vi "configuration UI.vi"() -> ()   [LabVIEW 2013, in "configuration tests.lvlib" / "TEST EDITOR.lvclass"]
uses:
  TEST EDITOR.lvclass
  <vilib>/NI/Configuration Framework/Node/NodeRef.ctl
  <vilib>/NI/Configuration Framework/Node/NISE_CEF_Node.lvclass
  <vilib>/NI/AMC/Message Queue.ctl
  <vilib>/NI/AMC/Message.ctl
  <vilib>/NI/Tools/Keyed Array/KeyedArray.ctl
  <vilib>/NI/Configuration Framework/Node/UserEventRef.ctl
  <vilib>/NI/Configuration Framework/Controls/EventCluster.ctl
  module/configuration/TEST CONFIGURATION.lvclass
  TEST EDITOR.lvclass/TEST EDITOR.ctl
  <vilib>/NI/Configuration Framework/serializable configuration/NISE_CEF_serializable configuration.lvclass/NISE_CEF_serializable configuration.ctl
  Configuration Editor/Classes/Engine Parent/Engine Parent Editor Node.lvclass
  module/configuration/TEST CONFIGURATION.lvclass/TEST CONFIGURATION.ctl
  module/configuration/gains.ctl
  Read sort_.vi
  module/configuration/Read state module configuration.vi
  Write sort_.vi
  <vilib>/NI/Configuration Framework/serializable configuration/Read UID.vi
  Configuration Editor/Classes/Module editor node/Read Module Configuration.vi
  <vilib>/Utility/LVClass/Get LV Class Name.vi
  <vilib>/NI/Configuration Framework/error generator/NISE_error generator.vi
  <vilib>/NI/Tag Bus Module Framework/module configuration/TBM module configuration.lvclass
  <vilib>/NI/Tag Bus Module Framework/channel/TBM channel.lvclass
  <vilib>/NI/Configuration Framework/NISE_CEF_TreeControl.lvlib
  <vilib>/NI/Tools/Keyed Array/Tools_KeyedArray.lvlib
  <vilib>/NI/AMC/AMC.lvlib
panel:
  in  "Tab Control":T1(tab)
  in  "delete":bool
  in  "add":bool
  in  "Result Tag":u16(ring)
  in  "PV Tag":u16(ring)
  in  "Setpoint Tag":u16(ring)
  in  "Functions":i32(listbox)
  in  "Function Name":string
  in  "Lower Limit":dbl=-100.0
  in  "Upper Limit":dbl=100.0
  in  "Ki":dbl
  in  "Kd":dbl
  in  "Kp":dbl
  in  "Output Tag":u16(ring)
  in  "Input Tag":u16(ring)
  in  "user event":T2
  in  "main queue":T3
  in  "node ref":T4
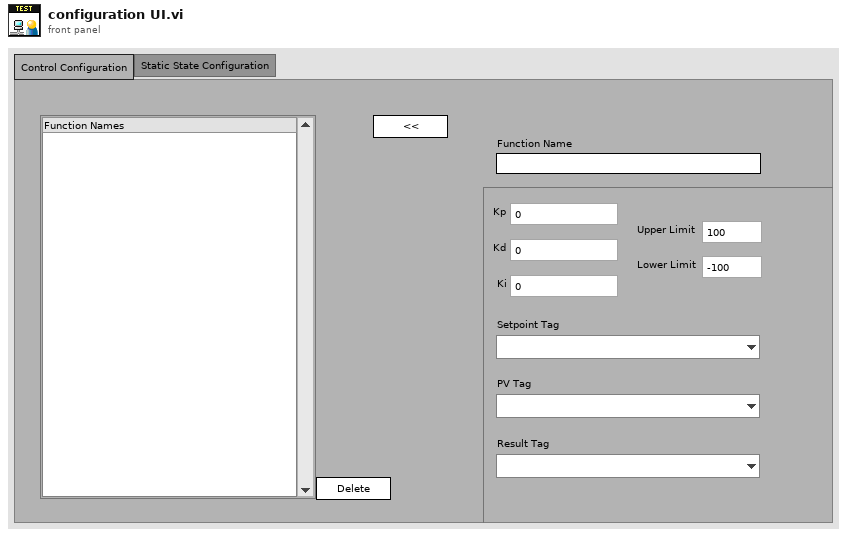
[diagram p1: front panel]
types:
  T1 = enum32{"Control Configuration", "Static State Configuration"}
  T2 = typedef "NISE_CEF_Node.lvclass/UserEventRef.ctl" = refnum<user-event>
  T3 = typedef "AMC.lvlib/Message Queue.ctl" = refnum<queue>
  T4 = typedef "NISE_CEF_Node.lvclass/NodeRef.ctl" = refnum<data-value>
  T5 = typedef "NISE_CEF_TreeControl.lvlib/EventCluster.ctl" = cluster{"command":string, "data":string}
  T6 = typedef "configuration tests.lvlib/TEST CONFIGURATION.lvclass/gains.ctl" = cluster{"Kp":dbl, "Ki":dbl, "Kd":dbl}
  T7 = typedef "user tag bus module configuration.lvclass/state module configuration.ctl" = cluster{"fixed input":refnum<class "TBM channel.lvclass">, "fixed output":refnum<class "TBM channel.lvclass">, "initial state":u8}
  T8 = typedef "configuration tests.lvlib/TEST CONFIGURATION.lvclass/control module configuration.ctl" = cluster{"name":string, "setpoint":refnum<class "TBM channel.lvclass">, "process variable":refnum<class "TBM channel.lvclass">, "output":refnum<class "TBM channel.lvclass">, "gains":T6, "output range":cluster{"output high":dbl, "output low":dbl}}
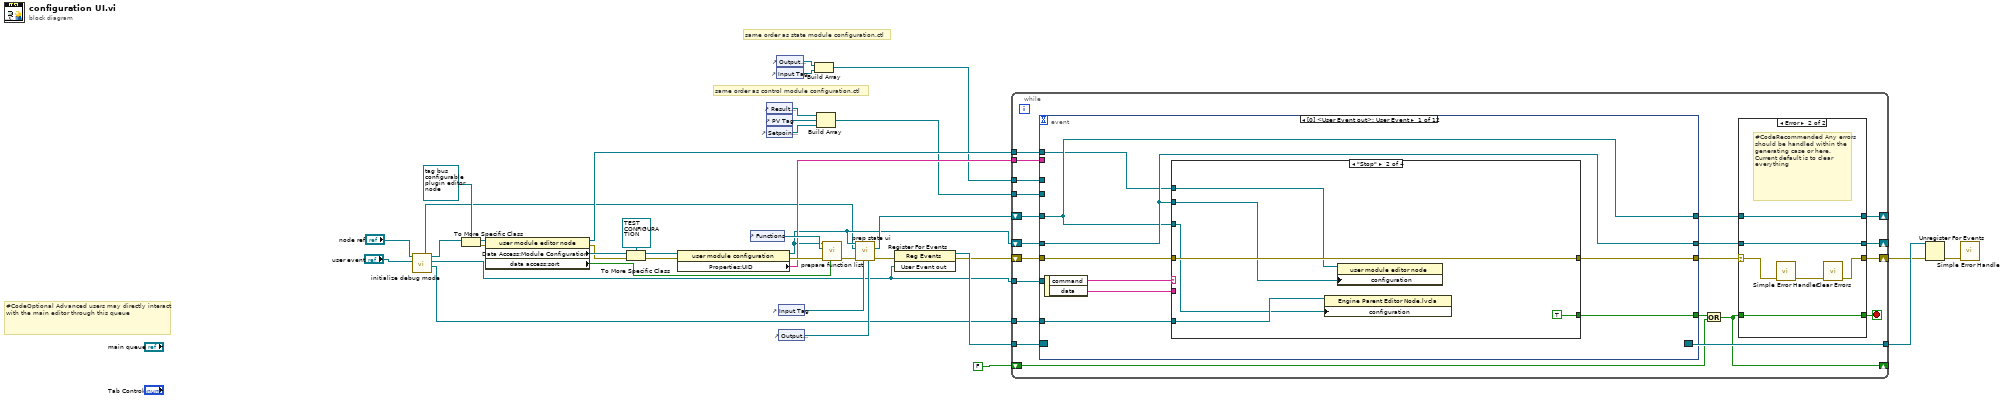
[diagram p0: block diagram]
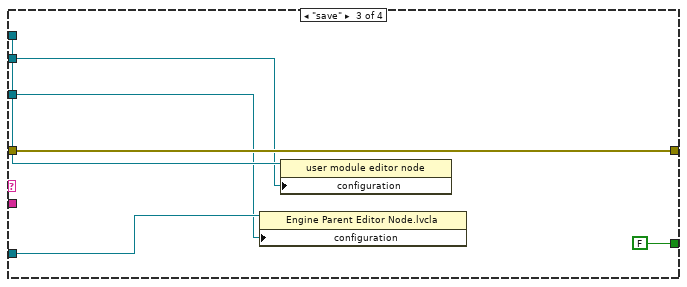
[diagram p4: hidden frame]
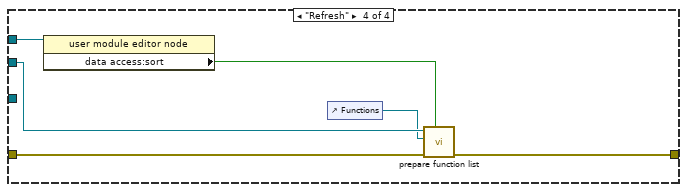
[diagram p5: hidden frame]
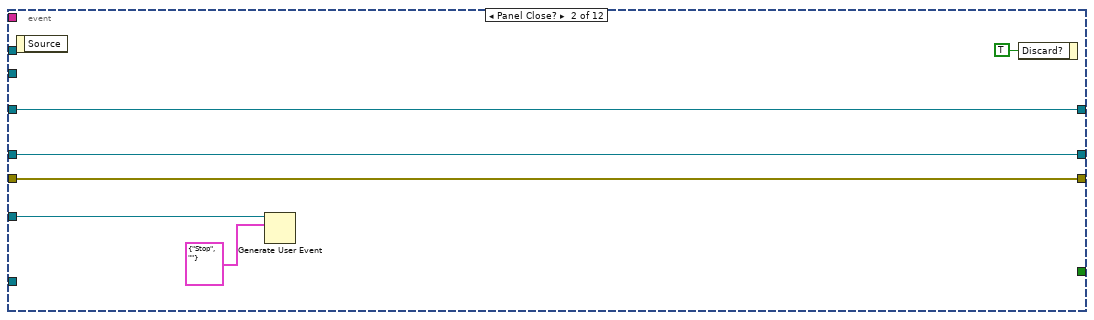
[diagram p6: hidden frame]
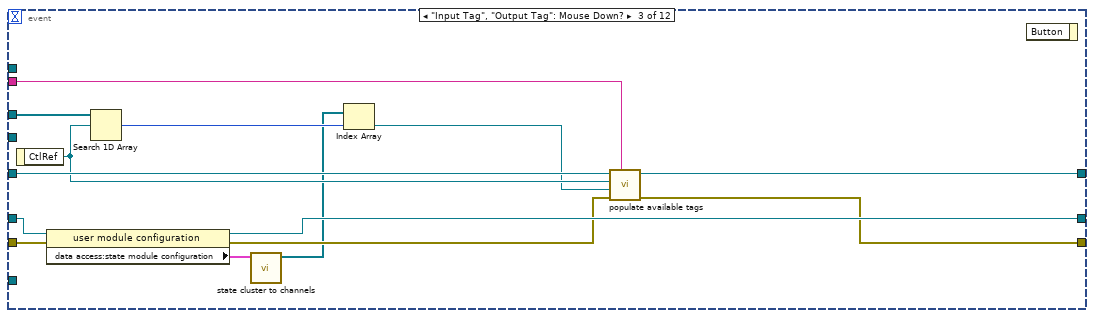
[diagram p7: hidden frame]
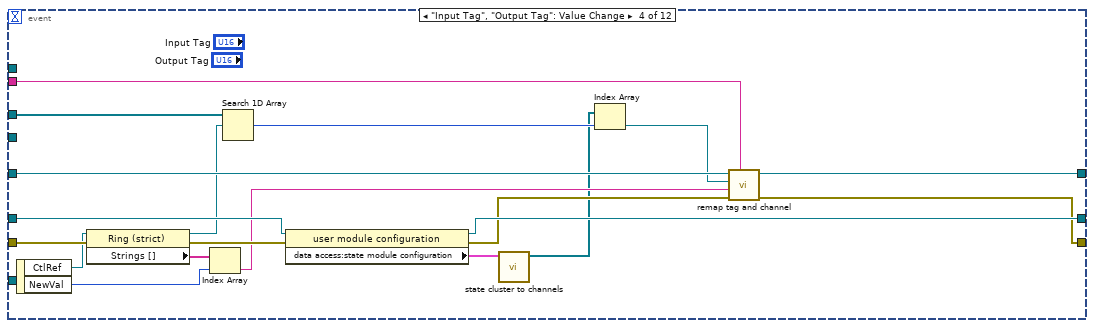
[diagram p8: hidden frame]
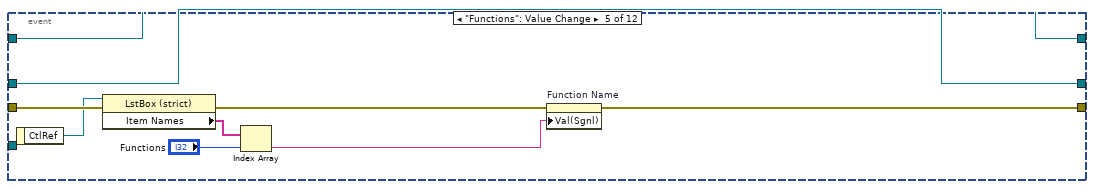
[diagram p9: hidden frame]
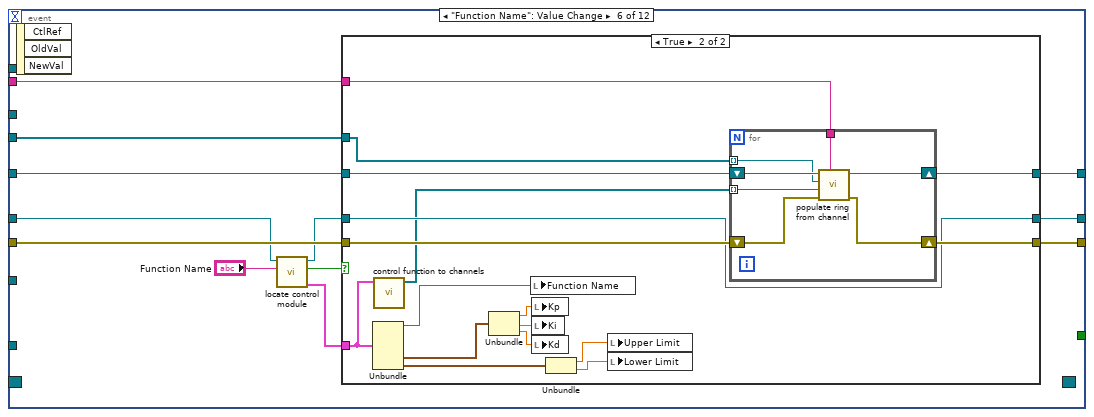
[diagram p10: hidden frame]
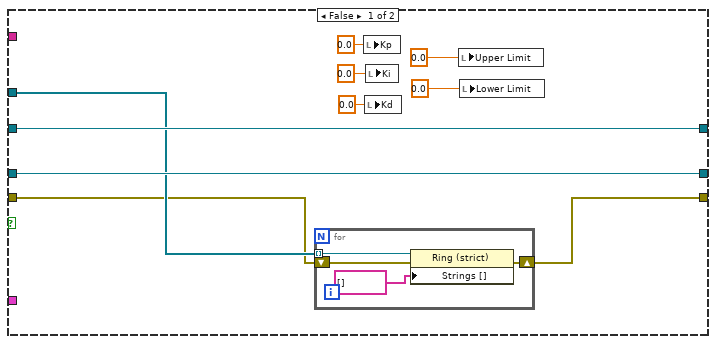
[diagram p11: hidden frame]
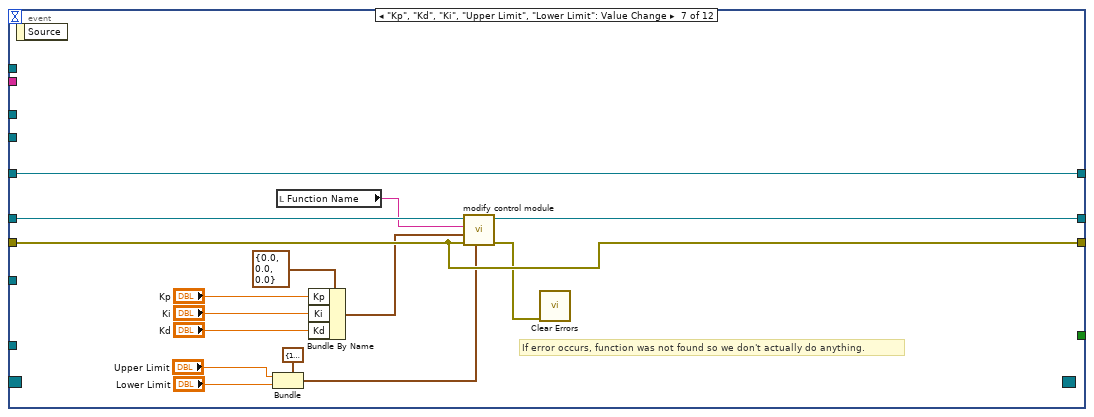
[diagram p12: hidden frame]
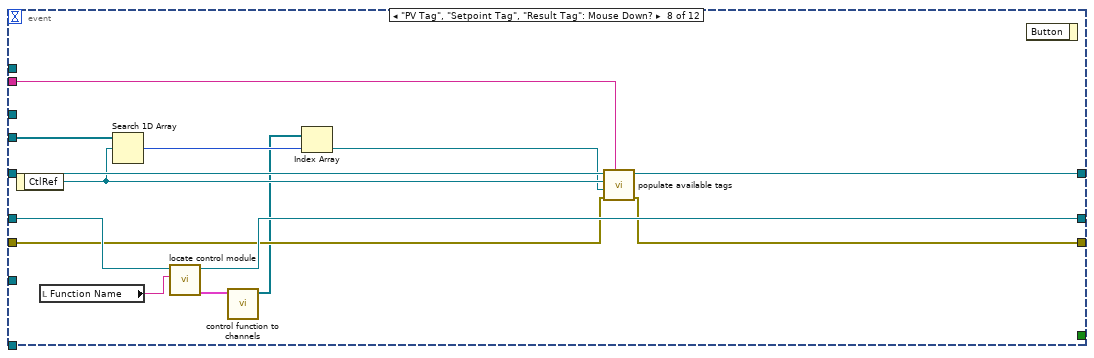
[diagram p13: hidden frame]
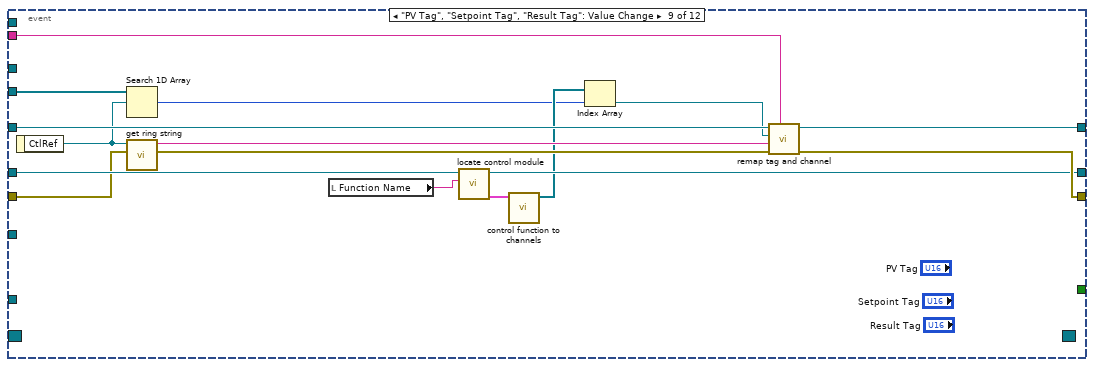
[diagram p14: hidden frame]
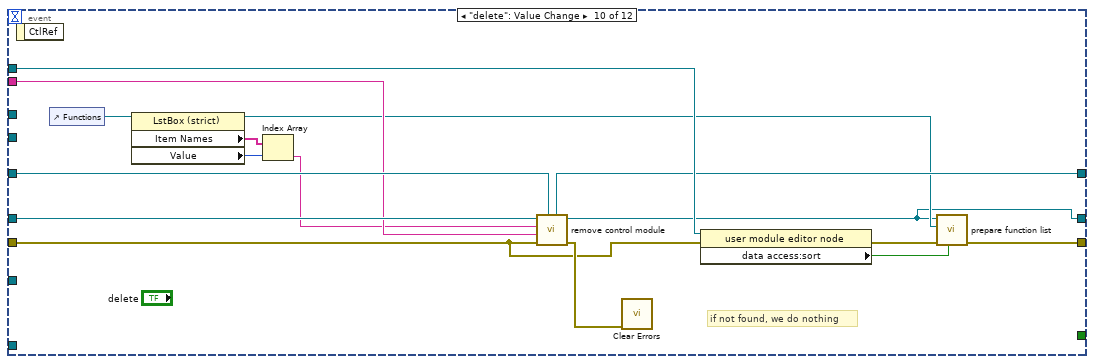
[diagram p15: hidden frame]
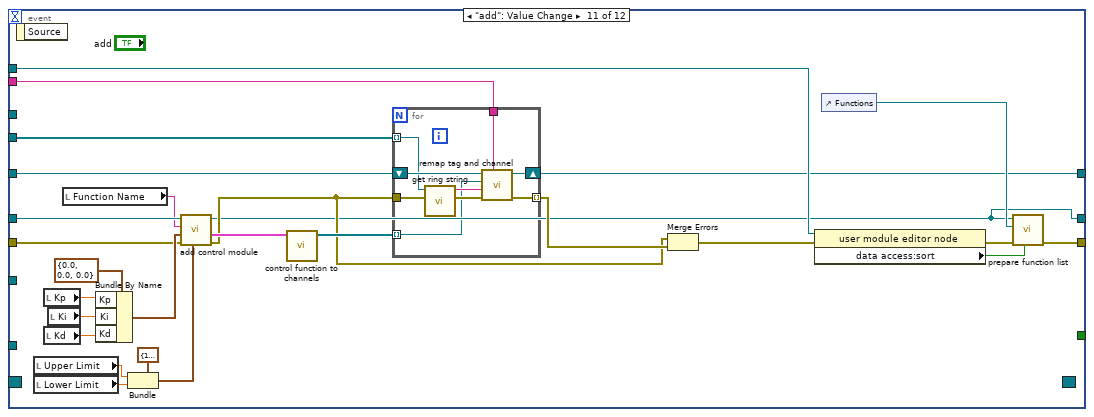
[diagram p16: hidden frame]
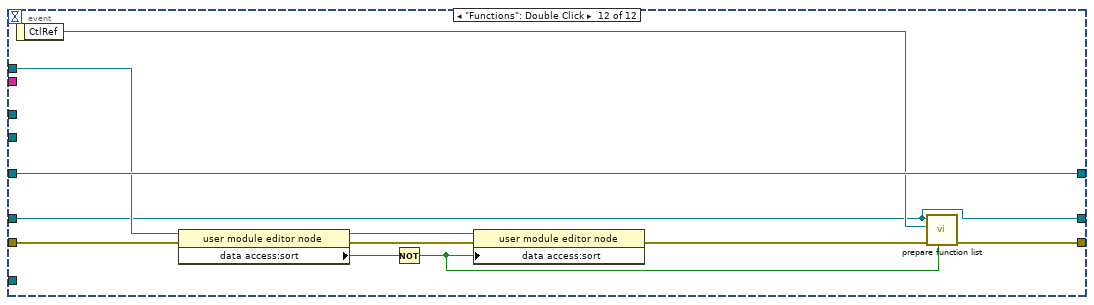
[diagram p17: hidden frame]
diagram:
  # "same order as control module configuration.ctl"
  # "same order as state module configuration.ctl"
  # "#CodeOptional Advanced users may directly interact with the main editor through this queue"
  n1 = call "initialize debug mode.vi"("User Event in"="user event", "editor node in"="node ref") -> ("engine"=w6:refnum<data-value>, "User Event out"=w1:T2, "editor node out"=w5:T4, "Engine Configuration"=w2:refnum<class "engine configuration.lvclass">)  [unwired: 6 in]
  n2 = To More Specific Class(target class=refnum<data-value> refnum ("data value reference"), reference=w5) -> (specific class reference=w31:refnum<data-value>, error out=w30:errorcluster)  [unwired: 1 in]
  n3 = property class="user module editor node"(reference=w31, error in=w30) -> (reference out=w16:refnum<data-value>, error out=w25:errorcluster, "Data Access:Module Configuration"=w29:refnum<class "TBM module configuration.lvclass">, "data access:sort"=w15:bool)
  n4 = To More Specific Class(target class=refnum<class "TEST CONFIGURATION.lvclass"> refnum ("user module configuration"), reference=w29, error in=w25) -> (specific class reference=w23:refnum<class "TEST CONFIGURATION.lvclass">, error out=w27:errorcluster)
  n5 = property class="user module configuration"(reference=w23, error in=w27) -> (reference out=w7:refnum<class "TEST CONFIGURATION.lvclass">, error out=w24:errorcluster, "Properties:UID"=w22:string)
  n6 = control-ref of="Functions"() -> (w26:refnum<vi>)
  n7 = control-ref of="Result Tag"() -> (w10:refnum<vi>)
  n8 = control-ref of="PV Tag"() -> (w12:refnum<vi>)
  n9 = control-ref of="Setpoint Tag"() -> (w11:refnum<vi>)
  n10 = control-ref of="Output Tag"() -> (w13:refnum<vi>)
  n11 = control-ref of="Input Tag"() -> (w14:refnum<vi>)
  n12 = control-ref of="Input Tag"() -> (w19:refnum<vi>)
  n13 = control-ref of="Output Tag"() -> (w18:refnum<vi>)
  n14 = Build Array(w13, w14) -> (w9:refnum<vi>[])
  n15 = Build Array(w10, w12, w11) -> (w8:refnum<vi>[])
  n16 = call "prepare function list.vi"("sort?"=w15, "error in"=w24, "Functions listbox"=w26, "configuration in"=w7) -> ("error out"=w20:errorcluster)  [unwired: 5 in]
  n17 = call "prep state ui.vi"("Output Tag"=w18, "Input Tag"=w19, "error in"=w20, "engine configuration in"=w2, "user tag bus module configuration in"=w7) -> ("error out"=w21:errorcluster, "engine configuration out"=w17:refnum<class "engine configuration.lvclass">)  [unwired: 5 in]
  n18 = register-events(error in=w21, w1) -> (reference out=w38:refnum<event-registration>, error out=w33:errorcluster)  [unwired: 1 in]
  n19 = while {
    tunnel: w38 -> [w59]
    tunnel: [w58] -> w37
    shift-right: [w51] -> w36
    shift-left: w33 -> [w57]
    shift-right: [w53] -> _
    shift-left: FALSE -> [w52]
    shift-right: [w48] -> _
    shift-left: w7 -> [w50]
    shift-right: [w45] -> _
    shift-left: w17 -> [w47]
    tunnel: w22 -> [w44]
    tunnel: w16 -> [w43]
    tunnel: w6 -> [w42]
    tunnel: w9 -> [w41]
    tunnel: w8 -> [w40]
    tunnel: w1 -> [w39]
    stop <- w55 stop-if-true
    n20 = event shown="[0] <User Event out>: User Event" {
      selector: w59 -> [_ _ _ _ _ _ _ _ _ _ _ _]
      dyn-events: [_ _ _ _ _ _ _ _ _ _ _ _] -> w58
      timeout: _ -> [_ _ _ _ _ _ _ _ _ _ _ _]
      tunnel: [w76 _ _ _ _ _ _ _ _ _ _ _] -> w54
      tunnel: [w77 w103 w113 w128 w137 w153 w209 w217 w238 w254 w283 w302] -> w56
      tunnel: w57 -> [w78 w103 w117 w136 w145 w157 w209 w218 w231 w251 w265 w301]
      tunnel: [w74 w102 w114 w130 w144 w154 w207 w223 w234 w241 w257 w293] -> w49
      tunnel: w50 -> [w74 w102 w115 w131 w144 w152 w210 w224 w235 w256 w275 w293]
      tunnel: w47 -> [w73 w101 w112 w133 w143 w155 w205 w221 w240 w248 w276 w303]
      tunnel: [w73 w101 w116 w129 w143 w156 w205 w220 w239 w247 w277 w303] -> w46
      tunnel: w44 -> [_ _ w111 w126 _ w148 _ w219 w237 w246 w278 _]
      tunnel: w43 -> [w72 _ _ _ _ _ _ _ _ w249 w279 w297]
      tunnel: w42 -> [w71 _ _ _ _ _ _ _ _ _ _ _]
      tunnel: w41 -> [_ _ w109 w124 _ _ _ _ _ _ _ _]
      tunnel: w40 -> [_ _ _ _ _ w146 _ w215 w230 _ w260 _]
      tunnel: w39 -> [_ w99 _ _ _ _ _ _ _ _ _ _]
      event User Event {
        n21 = event-data() -> ("command"=w75:string, "data"=w70:string)  [unwired: 1 in]
        n22 = case shown="\"Stop\"" w75 {
          tunnel: [_ TRUE FALSE _] -> w76
          tunnel: w71 -> [_ w84 w90 _]
          tunnel: w74 -> [_ w81 w86 w94]
          tunnel: w73 -> [_ w80 w87 _]
          tunnel: w78 -> [w79 w83 w89 w95]
          tunnel: [w79 w83 w89 w96] -> w77
          tunnel: w72 -> [_ w82 w88 w97]
          tunnel: w70 -> [_ _ _ _]
          frame Default {
          }
          frame "Stop" {
            n23 = property class="Engine Parent Editor Node.lvcla"(reference=w84, "configuration"=w80) -> ()  [unwired: 1 in, 2 out]
            n24 = property class="user module editor node"(reference=w82, "configuration"=w81) -> ()  [unwired: 1 in, 2 out]
          }
          frame "save" {
            n25 = property class="Engine Parent Editor Node.lvcla"(reference=w90, "configuration"=w87) -> ()  [unwired: 1 in, 2 out]
            n26 = property class="user module editor node"(reference=w88, "configuration"=w86) -> ()  [unwired: 1 in, 2 out]
          }
          frame "Refresh" {
            n27 = property class="user module editor node"(reference=w97) -> ("data access:sort"=w93:bool)  [unwired: 1 in, 2 out]
            n28 = control-ref of="Functions"() -> (w92:refnum<vi>)
            n29 = call "prepare function list.vi"("sort?"=w93, "error in"=w95, "Functions listbox"=w92, "configuration in"=w94) -> ("error out"=w96:errorcluster)  [unwired: 5 in]
          }
        }
      }
      event Panel Close? {
        n30 = event-data() -> ()  [unwired: 1 in, 1 out]
        n31 = Generate User Event(user event=w99, event data cluster=T5 {"command"="Stop", "data"=""} ("event data")) -> ()  [unwired: 2 in, 2 out]
        n32 = event-data("Discard?"=TRUE) -> ()  [unwired: 1 in, 1 out]
      }
      event "Input Tag", "Output Tag": Mouse Down? {
        n33 = event-data() -> ("CtlRef"=w108:refnum<vi>)  [unwired: 1 in]
        n34 = property class="user module configuration"(reference=w115, error in=w117) -> (reference out=w114:refnum<class "TEST CONFIGURATION.lvclass">, error out=w110:errorcluster, "data access:state module configuration"=w106:T7)
        n35 = Search 1D Array(1D array=w109, element=w108) -> (index of element=w107:i32)  [unwired: 1 in]
        n36 = call "state cluster to channels.vi"("state module configuration"=w106) -> ("channels"=w105:refnum<class "TBM channel.lvclass">[])  [unwired: 10 in]
        n37 = Index Array(array=w105, index=w107) -> (element=w104:refnum<class "TBM channel.lvclass">)
        n38 = call "populate available tags.vi"("instance id"=w111, "error in"=w110, "channel"=w104, "CtlRef"=w108, "engine configuration in"=w112) -> ("error out"=w113:errorcluster, "engine configuration out"=w116:refnum<class "engine configuration.lvclass">)  [unwired: 5 in]
        n39 = event-data() -> ()  [unwired: 2 in, 1 out]
      }
      event "Input Tag", "Output Tag": Value Change {
        n40 = event-data() -> ("CtlRef"=w135:refnum<vi>, "NewVal"=w122:u16)  [unwired: 1 in]
        n41 = property on="Property Node" class="Ring (strict)"(reference=w135, error in=w136) -> (reference out=w123:refnum<vi>, error out=w132:errorcluster, "Strings []"=w134:string[])
        n42 = Index Array(array=w134, index=w122) -> (element=w125:string)
        n43 = Search 1D Array(1D array=w124, element=w123) -> (index of element=w120:i32)  [unwired: 1 in]
        n44 = property class="user module configuration"(reference=w131, error in=w132) -> (reference out=w130:refnum<class "TEST CONFIGURATION.lvclass">, error out=w127:errorcluster, "data access:state module configuration"=w121:T7)
        n45 = call "state cluster to channels.vi"("state module configuration"=w121) -> ("channels"=w119:refnum<class "TBM channel.lvclass">[])  [unwired: 10 in]
        n46 = Index Array(array=w119, index=w120) -> (element=w118:refnum<class "TBM channel.lvclass">)
        n47 = call "remap tag and channel.vi"("instance id"=w126, "error in"=w127, "tag name"=w125, "channel"=w118, "engine configuration in"=w133) -> ("error out"=w128:errorcluster, "engine configuration out"=w129:refnum<class "engine configuration.lvclass">)  [unwired: 5 in]
      }
      event "Functions": Value Change {
        n48 = event-data() -> ("CtlRef"=w142:refnum<vi>)  [unwired: 1 in]
        n49 = property class="LstBox (strict)"(reference=w142, error in=w145) -> (error out=w138:errorcluster, "Item Names"=w141:string[])  [unwired: 1 out]
        n50 = Index Array(array=w141, index="Functions") -> (element=w139:string)
        n51 = property on="Function Name" class="Str"(error in=w138, "Val(Sgnl)"=w139) -> (error out=w137:errorcluster)  [unwired: 1 in, 1 out]
      }
      event "Function Name": Value Change {
        n52 = event-data() -> ()  [unwired: 1 in, 3 out]
        n53 = call "locate control module.vi"("name"="Function Name", "user module configuration in"=w152) -> ("module duplicate"=w149:T8, "found"=w150:bool, "user module configuration out"=w151:refnum<class "TEST CONFIGURATION.lvclass">)  [unwired: 6 in, 1 out]
        n54 = case shown="True" w150 {
          tunnel: [w167 w180] -> w156
          tunnel: w155 -> [w167 w178]
          tunnel: w151 -> [w166 w175]
          tunnel: [w166 w175] -> w154
          tunnel: w157 -> [w164 w177]
          tunnel: [w163 w176] -> w153
          tunnel: w149 -> [_ w174]
          tunnel: w148 -> [_ w179]
          tunnel: w146 -> [w165 w173]
          frame False {
            n55 = for {
              shift-right: [w171] -> w163
              shift-left: w164 -> [w170]
              tunnel: w165 -> [w168] mode=indexing
              n56 = property on="Property Node" class="Ring (strict)"(reference=w168, error in=w170, "Strings []"=string[] []) -> (error out=w171:errorcluster)  [unwired: 1 out]
            }
            n57 = local write "Kp"(0.0 ("Kp")) -> ()
            n58 = local write "Kd"(0.0 ("Kp")) -> ()
            n59 = local write "Ki"(0.0 ("Kp")) -> ()
            n60 = local write "Upper Limit"(0.0 ("Kp")) -> ()
            n61 = local write "Lower Limit"(0.0 ("Kp")) -> ()
          }
          frame True {
            n62 = Unbundle(w174) -> ("name"=w181:string, "gains"=w188:T6, "output range"=w187:cluster{"output high":dbl, "output low":dbl})  [unwired: 3 out]
            n63 = call "control function to channels.vi"("control module configuration"=w174) -> ("channels"=w172:refnum<class "TBM channel.lvclass">[])  [unwired: 10 in]
            n64 = Unbundle(w188) -> ("Kp"=w182:dbl, "Ki"=w183:dbl, "Kd"=w184:dbl)
            n65 = local write "Function Name"(w181) -> ()
            n66 = local write "Kp"(w182) -> ()
            n67 = local write "Ki"(w183) -> ()
            n68 = local write "Kd"(w184) -> ()
            n69 = Unbundle(w187) -> ("output high"=w185:dbl, "output low"=w186:dbl)
            n70 = local write "Upper Limit"(w185) -> ()
            n71 = local write "Lower Limit"(w186) -> ()
            n72 = for {
              tunnel: w179 -> [w194]
              shift-right: [w195] -> w180
              shift-left: w178 -> [w193]
              shift-right: [w191] -> w176
              shift-left: w177 -> [w192]
              tunnel: w173 -> [w190] mode=indexing
              tunnel: w172 -> [w189] mode=indexing
              n73 = call "populate ring from channel.vi"("instance id"=w194, "error in"=w192, "channel"=w189, "ring"=w190, "engine configuration in"=w193) -> ("error out"=w191:errorcluster, "engine configuration out"=w195:refnum<class "engine configuration.lvclass">)  [unwired: 4 in, 1 out]
            }
          }
        }
      }
      event "Kp", "Kd", "Ki", "Upper Limit", "Lower Limit": Value Change {
        # "If error occurs, function was not found so we don't actually do anything."
        n74 = event-data() -> ()  [unwired: 1 in, 1 out]
        n75 = Bundle(cluster=cluster{"output high":dbl, "output low":dbl} {"output high"=100.0, "output low"=-100.0} ("output range"), "output high"="Upper Limit", "output low"="Lower Limit") -> (w201:cluster{"output high":dbl, "output low":dbl})
        n76 = local read "Function Name"() -> (w206:string)
        n77 = Bundle By Name(cluster=T6 {"Kp"=0.0, "Ki"=0.0, "Kd"=0.0} ("gains"), "Kp"="Kp", "Ki"="Ki", "Kd"="Kd") -> (w196:T6)
        n78 = call "modify control module.vi"("output range"=w201, "error in"=w209, "gains"=w196, "name"=w206, "user module configuration in"=w210) -> ("error out"=w208:errorcluster, "user module configuration out"=w207:refnum<class "TEST CONFIGURATION.lvclass">)  [unwired: 5 in]
        n79 = call <vilib>:"Clear Errors.vi"("error in (no error)"=w208) -> ()  [unwired: 6 in, 1 out]
      }
      event "PV Tag", "Setpoint Tag", "Result Tag": Mouse Down? {
        n80 = event-data() -> ("CtlRef"=w214:refnum<vi>)  [unwired: 1 in]
        n81 = local read "Function Name"() -> (w222:string)
        n82 = Search 1D Array(1D array=w215, element=w214) -> (index of element=w213:i32)  [unwired: 1 in]
        n83 = call "locate control module.vi"("name"=w222, "user module configuration in"=w224) -> ("module duplicate"=w216:T8, "user module configuration out"=w223:refnum<class "TEST CONFIGURATION.lvclass">)  [unwired: 6 in, 2 out]
        n84 = call "control function to channels.vi"("control module configuration"=w216) -> ("channels"=w212:refnum<class "TBM channel.lvclass">[])  [unwired: 10 in]
        n85 = Index Array(array=w212, index=w213) -> (element=w211:refnum<class "TBM channel.lvclass">)
        n86 = call "populate available tags.vi"("instance id"=w219, "error in"=w218, "channel"=w211, "CtlRef"=w214, "engine configuration in"=w221) -> ("error out"=w217:errorcluster, "engine configuration out"=w220:refnum<class "engine configuration.lvclass">)  [unwired: 5 in]
        n87 = event-data() -> ()  [unwired: 2 in, 1 out]
      }
      event "PV Tag", "Setpoint Tag", "Result Tag": Value Change {
        n88 = event-data() -> ("CtlRef"=w229:refnum<vi>)  [unwired: 1 in]
        n89 = Search 1D Array(1D array=w230, element=w229) -> (index of element=w226:i32)  [unwired: 1 in]
        n90 = call "get ring string.vi"("error in"=w231, "Ring in"=w229) -> ("error out"=w232:errorcluster, "String"=w233:string)  [unwired: 8 in]
        n91 = local read "Function Name"() -> (w236:string)
        n92 = call "locate control module.vi"("name"=w236, "user module configuration in"=w235) -> ("module duplicate"=w228:T8, "user module configuration out"=w234:refnum<class "TEST CONFIGURATION.lvclass">)  [unwired: 6 in, 2 out]
        n93 = call "control function to channels.vi"("control module configuration"=w228) -> ("channels"=w227:refnum<class "TBM channel.lvclass">[])  [unwired: 10 in]
        n94 = Index Array(array=w227, index=w226) -> (element=w225:refnum<class "TBM channel.lvclass">)
        n95 = call "remap tag and channel.vi"("instance id"=w237, "error in"=w232, "tag name"=w233, "channel"=w225, "engine configuration in"=w240) -> ("error out"=w238:errorcluster, "engine configuration out"=w239:refnum<class "engine configuration.lvclass">)  [unwired: 5 in]
      }
      event "delete": Value Change {
        # "if not found, we do nothing"
        n96 = event-data() -> ()  [unwired: 1 in, 1 out]
        n97 = control-ref of="Functions"() -> (w250:refnum<vi>)
        n98 = property class="LstBox (strict)"(reference=w250) -> (reference out=w245:refnum<vi>, "Item Names"=w244:string[], "Value"=w243:i32)  [unwired: 1 in, 1 out]
        n99 = Index Array(array=w244, index=w243) -> (element=w242:string)
        n100 = call "remove control module.vi"("engine in"=w248, "error in"=w251, "owner id"=w246, "name"=w242, "user module configuration in"=w256) -> ("error out"=w255:errorcluster, "user module configuration out"=w241:refnum<class "TEST CONFIGURATION.lvclass">, "engine out"=w247:refnum<class "engine configuration.lvclass">)  [unwired: 4 in]
        n101 = call <vilib>:"Clear Errors.vi"("error in (no error)"=w255) -> ()  [unwired: 6 in, 1 out]
        n102 = property class="user module editor node"(reference=w249, error in=w251) -> (error out=w253:errorcluster, "data access:sort"=w252:bool)  [unwired: 1 out]
        n103 = call "prepare function list.vi"("sort?"=w252, "error in"=w253, "Functions listbox"=w245, "configuration in"=w241) -> ("error out"=w254:errorcluster)  [unwired: 5 in]
      }
      event "add": Value Change {
        n104 = event-data() -> ()  [unwired: 1 in, 1 out]
        n105 = local read "Upper Limit"() -> (w274:dbl)
        n106 = local read "Lower Limit"() -> (w273:dbl)
        n107 = local read "Kp"() -> (w268:dbl)
        n108 = local read "Kd"() -> (w270:dbl)
        n109 = local read "Ki"() -> (w269:dbl)
        n110 = local read "Function Name"() -> (w264:string)
        n111 = Bundle By Name(cluster=T6 {"Kp"=0.0, "Ki"=0.0, "Kd"=0.0} ("gains"), "Kp"=w268, "Ki"=w269, "Kd"=w270) -> (w266:T6)
        n112 = Bundle(cluster=cluster{"output high":dbl, "output low":dbl} {"output high"=100.0, "output low"=-100.0} ("output range"), "output high"=w274, "output low"=w273) -> (w271:cluster{"output high":dbl, "output low":dbl})
        n113 = call "add control module.vi"("output range"=w271, "error in"=w265, "gains"=w266, "name"=w264, "user module configuration in"=w275) -> ("error out"=w258:errorcluster, "generated control module"=w262:T8, "user module configuration out"=w257:refnum<class "TEST CONFIGURATION.lvclass">)  [unwired: 3 in, 1 out]
        n114 = call "control function to channels.vi"("control module configuration"=w262) -> ("channels"=w261:refnum<class "TBM channel.lvclass">[])  [unwired: 10 in]
        n115 = for {
          tunnel: w278 -> [w292]
          shift-right: [w291] -> w277
          shift-left: w276 -> [w290]
          tunnel: w261 -> [w285] mode=indexing
          tunnel: w260 -> [w284] mode=indexing
          tunnel: w258 -> [w287]
          tunnel: [w286] -> w263 mode=indexing
          n116 = call "get ring string.vi"("error in"=w287, "Ring in"=w284) -> ("error out"=w289:errorcluster, "String"=w288:string)  [unwired: 8 in]
          n117 = call "remap tag and channel.vi"("instance id"=w292, "error in"=w289, "tag name"=w288, "channel"=w285, "engine configuration in"=w290) -> ("error out"=w286:errorcluster, "engine configuration out"=w291:refnum<class "engine configuration.lvclass">)  [unwired: 5 in]
        }
        n118 = Merge Errors(w258, w263) -> (w259:errorcluster)
        n119 = property class="user module editor node"(reference=w279, error in=w259) -> (error out=w282:errorcluster, "data access:sort"=w281:bool)  [unwired: 1 out]
        n120 = control-ref of="Functions"() -> (w280:refnum<vi>)
        n121 = call "prepare function list.vi"("sort?"=w281, "error in"=w282, "Functions listbox"=w280, "configuration in"=w257) -> ("error out"=w283:errorcluster)  [unwired: 5 in]
      }
      event "Functions": Double Click {
        n122 = event-data() -> ("CtlRef"=w300:refnum<vi>)  [unwired: 1 in]
        n123 = property class="user module editor node"(reference=w297, error in=w301) -> (reference out=w296:refnum<data-value>, error out=w298:errorcluster, "data access:sort"=w295:bool)
        n124 = Not(x=w295) -> (.not. x?=w294:bool)
        n125 = property class="user module editor node"(reference=w296, error in=w298, "data access:sort"=w294) -> (error out=w299:errorcluster)  [unwired: 1 out]
        n126 = call "prepare function list.vi"("sort?"=w294, "error in"=w299, "Functions listbox"=w300, "configuration in"=w293) -> ("error out"=w302:errorcluster)  [unwired: 5 in]
      }
    }
    n127 = Or(x=w54, y=w52) -> (x .or. y?=w53:bool)
    n128 = case shown="Error" w56 {
      selector: w56 -> [w62 w68]
      tunnel: [w63 w69] -> w55
      tunnel: w53 -> [w63 w69]
      tunnel: [w62 w66] -> w51
      tunnel: w49 -> [w61 w65]
      tunnel: [w61 w65] -> w48
      tunnel: w46 -> [w60 w64]
      tunnel: [w60 w64] -> w45
      frame No Error {
      }
      frame Error {
        # "#CodeRecommended Any errors should be handled within the generating case or here. Current default is to clear everything"
        n129 = call <vilib>:"Simple Error Handler.vi"("error in (no error)"=w68) -> ("error out"=w67:errorcluster)  [unwired: 4 in, 4 out]
        n130 = call <vilib>:"Clear Errors.vi"("error in (no error)"=w67) -> ("error out"=w66:errorcluster)  [unwired: 6 in]
      }
    }
  }
  n131 = Unregister For Events(event registration refnum=w37, error in=w36) -> (error out=w32:errorcluster)
  n132 = call <vilib>:"Simple Error Handler.vi"("error in (no error)"=w32) -> ()  [unwired: 4 in, 5 out]
